vi "蓝牙串口接受.vi"() -> ()   [LabVIEW 2023]
uses:
  <vilib>/Instr/_visa.llb/VISA Flush IO Buffer Mask.ctl
  <vilib>/Instr/_visa.llb/VISA Configure Serial Port (Instr).vi
panel:
  out "同道2波形":u32(graph)
  out "通道1波形":u32(graph)
  in  "write_buffer":string
  in  "发送按钮":bool
  out "ReadBuffer":string
  out "读取返回数":u32
  in  "serial":refnum<visa-resource-name> caption="VISA资源名称"
  in  "串口开关":bool
  out "串口状态":bool
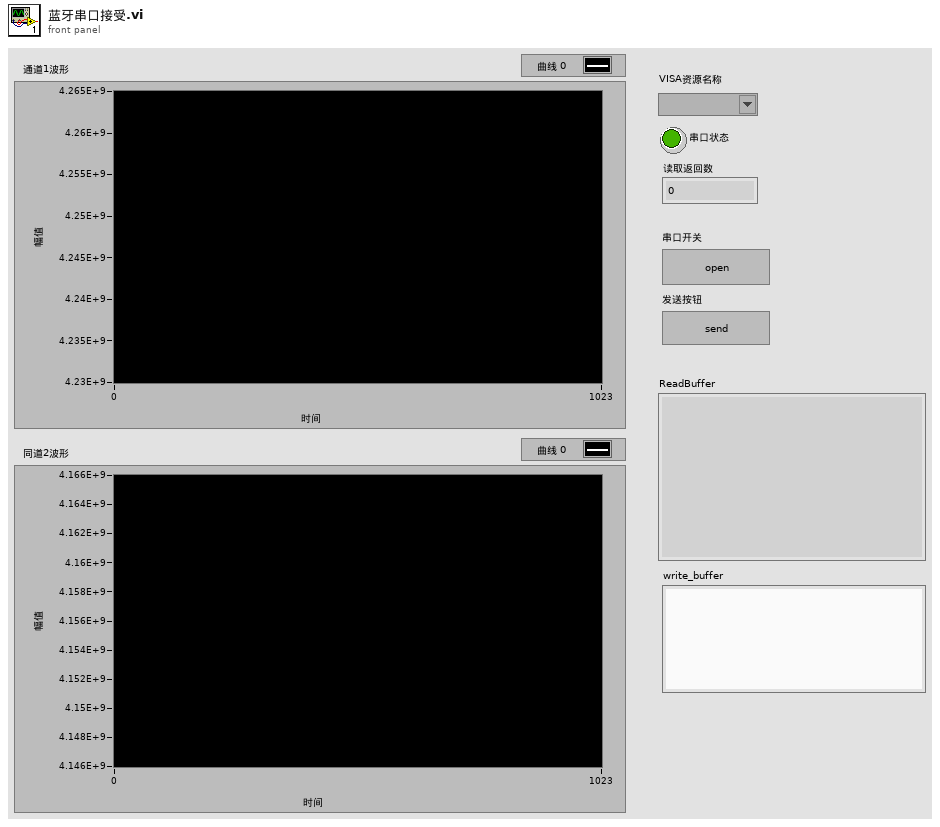
[diagram p1: front panel]
types:
  T1 = enum16{"nohead", "get_BB", "get_AA", "get_crc", "get_cnt"}
  T2 = cluster{"rx_finish":bool, "data_len":u8, "data":u8[], "head":enum16{"nohead", "get_BB", "get_AA", "get_crc", "get_cnt"}, "CRC":u8, "cnt":u8, "rx_len":u8}
  T3 = typedef "状态机控件.ctl" = enum16{"init_state", "main_state", "uart_receive_state", "stop_state"}
  T4 = typedef "VISA Flush IO Buffer Mask.ctl" = u16
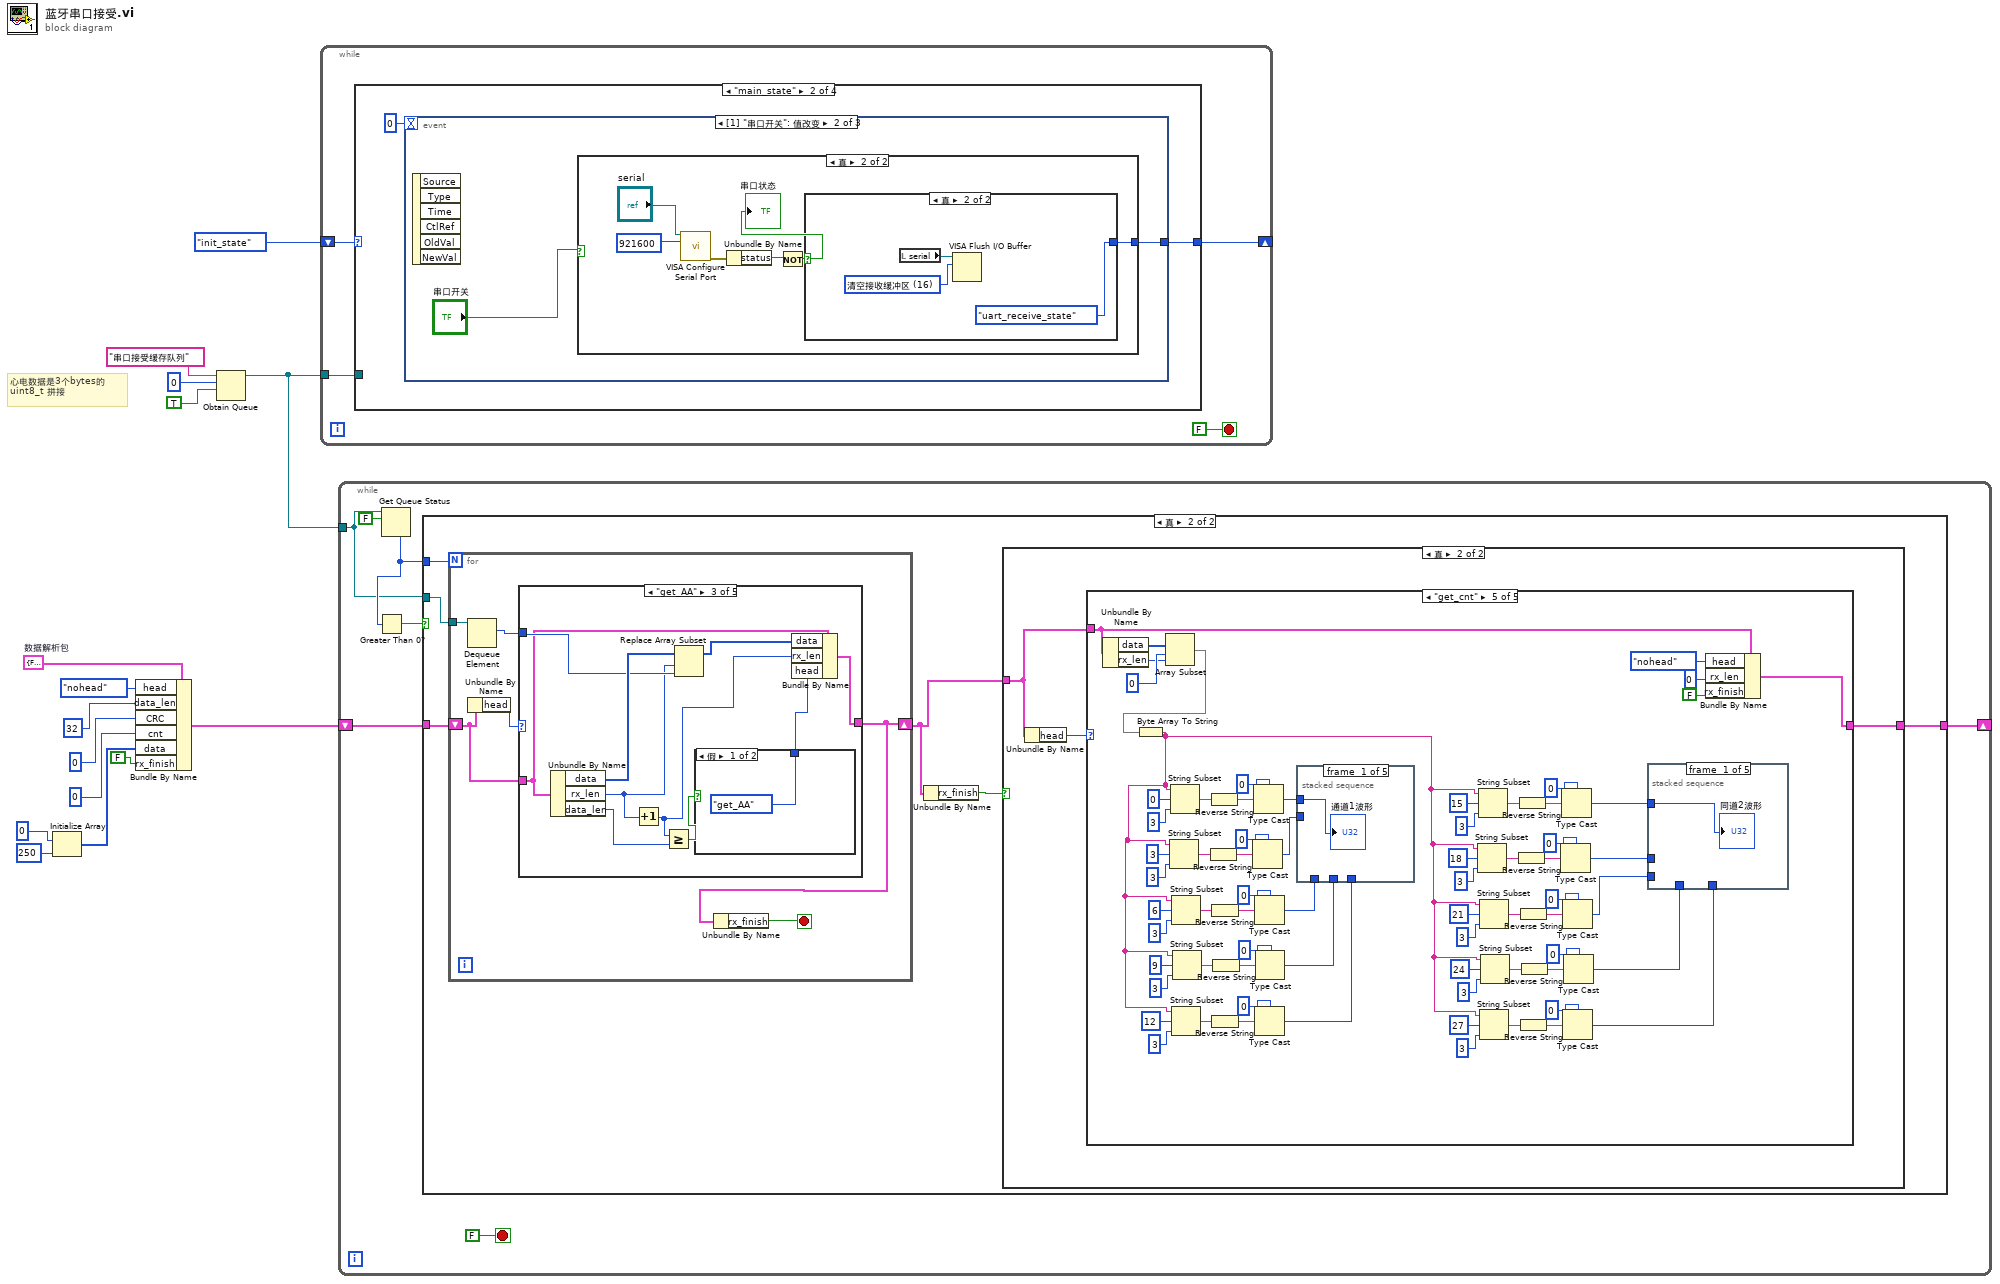
[diagram p0: block diagram]
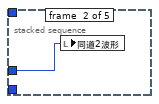
[diagram p8: hidden frame]
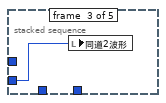
[diagram p9: hidden frame]
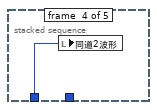
[diagram p10: hidden frame]
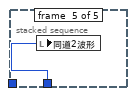
[diagram p11: hidden frame]
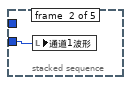
[diagram p12: hidden frame]
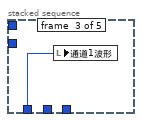
[diagram p13: hidden frame]
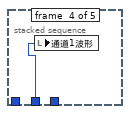
[diagram p14: hidden frame]
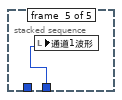
[diagram p15: hidden frame]
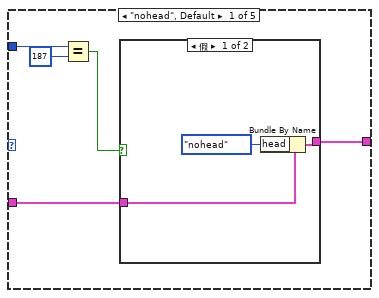
[diagram p16: hidden frame]
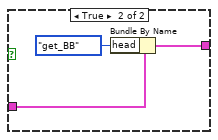
[diagram p17: hidden frame]
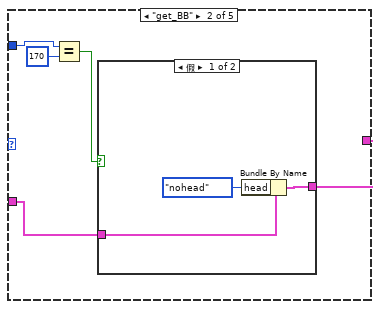
[diagram p18: hidden frame]
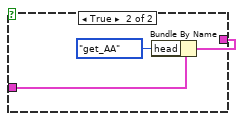
[diagram p19: hidden frame]
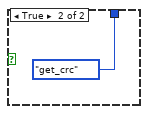
[diagram p20: hidden frame]
diagram:
  w11 = T2 {"rx_finish"=FALSE, "data_len"=0, "data"=[], "head"=enum."nohead", "CRC"=0, "cnt"=0, "rx_len"=0}  # 数据解析包
  # "心电数据是3个bytes的\nuint8_t 拼接"
  n1 = Initialize Array(u8 0 ("元素"), 250 ("维数大小")) -> (w4:u8[])
  n2 = Bundle By Name(cluster=w11, "head"=T1."nohead", "data_len"=u8 32, "CRC"=u8 0, "cnt"=u8 0 ("data_cnt"), "data"=w4, "rx_finish"=FALSE) -> (w10:T2)
  n3 = Obtain Queue(name (unnamed)="串口接受缓存队列" ("名称（未命名）"), element data type=u8 0, create if not found? (T)=TRUE ("如未找到则创建？(T)")) -> (queue out=w2:refnum<queue>)  [unwired: 2 in, 2 out]
  n4 = while {
    shift-right: [w19] -> _
    shift-left: 状态机控件."init_state" ("枚举") -> [w18]
    tunnel: w2 -> [w17]
    stop <- FALSE stop-if-true
    n5 = case shown="\"main_state\"" w18 {
      tunnel: [状态机控件."main_state" ("枚举") w27 w62 状态机控件."stop_state" ("枚举")] -> w19
      tunnel: w17 -> [_ _ w57 _]
      frame "init_state", Default {
        n6 = local write "write_buffer"("" ("write_buffer")) -> ()
        n7 = local write "ReadBuffer"("" ("ReadBuffer")) -> ()
        n8 = local write "串口开关"(FALSE ("串口状态")) -> ()
        n9 = local write "串口状态"(FALSE ("串口状态")) -> ()
        n10 = global write "全局变量1.vi" "while开关"(FALSE ("全局变量while开关")) -> ()
      }
      frame "main_state" {
        n11 = event shown="[1] \"串口开关\": 值改变" {
          selector: _ -> [_ _ _]
          dyn-events: _ -> [_ _ _]
          timeout: 0 -> [_ _ _]
          tunnel: [w29 w32 w50] -> w27
          event Timeout {
            n12 = event-data() -> ()  [unwired: 1 in, 3 out]
            n13 = local read "串口状态"() -> (w28:bool)
            n14 = case shown="假" w28 {
              tunnel: [状态机控件."main_state" ("枚举") 状态机控件."uart_receive_state" ("枚举")] -> w29
              frame False {
              }
              frame True {
              }
            }
          }
          event "串口开关": Value Change {
            n15 = event-data() -> ()  [unwired: 1 in, 6 out]
            n16 = case shown="真" "串口开关" {
              tunnel: [状态机控件."main_state" ("枚举") w37] -> w32
              frame False {
                # "关闭串口"
                n17 = local write "串口状态"(FALSE ("串口状态")) -> ()
                n18 = local read "serial"() -> (w35:refnum<visa-resource-name>)
                n19 = VISA Close(VISA resource name=w35) -> ()  [unwired: 1 in, 1 out]
              }
              frame True {
                n20 = call-poly "VISA Configure Serial Port"("VISA resource name"="serial", "baud rate (9600)"=u32 921600) -> ("error out"=w40:errorcluster)  [unwired: 12 in, 1 out]
                n21 = Unbundle By Name(w40) -> ("status"=w39:bool)
                n22 = Not(x=w39) -> (.not. x?=w38:bool)
                "串口状态" <- w38
                n23 = case shown="真" w38 {
                  tunnel: [状态机控件."main_state" ("枚举") 状态机控件."uart_receive_state" ("枚举")] -> w37
                  frame False {
                    n24 = local write "串口开关"(FALSE ("串口状态")) -> ()
                    n25 = One Button Dialog(message="串口打开失败" ("消息")) -> ()  [unwired: 1 in, 1 out]
                  }
                  frame True {
                    w46 = T4 16 items=["清空接收缓冲区"=16, "向设备写入传输缓冲区"=32, "清空接收缓冲区（无I/O）"=64, "清空传输缓冲区"=128] ("Mask")
                    n26 = local read "serial"() -> (w47:refnum<visa-resource-name>)
                    n27 = VISA Flush I/O Buffer(VISA resource name=w47, mask (16)=w46) -> ()  [unwired: 1 in, 2 out]
                  }
                }
              }
            }
          }
          event "发送按钮": Value Change {
            n28 = event-data() -> ()  [unwired: 1 in, 6 out]
            n29 = local read "串口状态"() -> (w49:bool)
            n30 = case shown="真" w49 {
              tunnel: [状态机控件."main_state" ("枚举") 状态机控件."uart_receive_state" ("枚举")] -> w50
              frame False {
                n31 = One Button Dialog(message="打开串口后在发送" ("消息")) -> ()  [unwired: 1 in, 1 out]
              }
              frame True {
                n32 = global write "全局变量1.vi" "while开关"(FALSE ("while开关")) -> ()
                n33 = local read "serial"() -> (w56:refnum<visa-resource-name>)
                n34 = VISA Write(VISA resource name=w56, write buffer="write_buffer") -> ()  [unwired: 1 in, 3 out]
              }
            }
          }
        }
      }
      frame "uart_receive_state" {
        n35 = local read "serial"() -> (w58:refnum<visa-resource-name>)
        n36 = property class="Instr"(reference=w58) -> (reference out=w60:refnum<visa-resource-name>, "Serial Settings:Number of Bytes at Serial Port"=w59:u32)  [unwired: 1 in, 1 out]
        n37 = Greater Than 0?(x=w59) -> (x > 0?=w61:bool)
        n38 = case shown="真" w61 {
          tunnel: [状态机控件."main_state" ("枚举") 状态机控件."main_state" ("枚举")] -> w62
          tunnel: w60 -> [_ w69]
          tunnel: w59 -> [_ w68]
          tunnel: w57 -> [_ w64]
          frame False {
          }
          frame True {
            # "注意点：for循环无法使用数组\n记住要关闭隧道索引"
            n39 = VISA Read(VISA resource name=w69, byte count=w68) -> (read buffer=w67:string)  [unwired: 1 in, 3 out]
            "ReadBuffer" <- w67
            n40 = String To Byte Array(string=w67) -> (unsigned byte array=w65:u8[])
            n41 = Array Size(array=w65) -> (size(s)=w66:i32)
            n42 = for {
              N: w66 -> [_]
              tunnel: w65 -> [w74]
              tunnel: w64 -> [w72]
              i -> [w73]
              # "队列数据通信 - > 队列操作\n\n先将串口读取到的数据存入队列"
              n43 = Index Array(array=w74, index=w73) -> (element=w71:u8)
              n44 = Enqueue Element(queue=w72, element=w71) -> ()  [unwired: 2 in, 3 out]
            }
            "读取返回数" <- w68
          }
        }
      }
      frame "stop_state" {
      }
    }
  }
  n45 = while {
    shift-right: [w78] -> _
    shift-left: w10 -> [w79]
    tunnel: w2 -> [w80]
    stop <- FALSE stop-if-true
    n46 = Get Queue Status(queue=w80, return elements? (F)=FALSE ("返回元素？(F)")) -> (# elements in queue=w81:i32)  [unwired: 1 in, 7 out]
    n47 = Greater Than 0?(x=w81) -> (x > 0?=w82:bool)
    n48 = case shown="真" w82 {
      tunnel: w81 -> [_ w89]
      tunnel: w80 -> [_ w88]
      tunnel: w79 -> [w83 w87]
      tunnel: [w83 w85] -> w78
      frame False {
      }
      frame True {
        n49 = for {
          N: w89 -> [_]
          tunnel: w88 -> [w183]
          shift-right: [w179] -> w84
          shift-left: w87 -> [w180]
          stop <- w178 stop-if-true
          n50 = Dequeue Element(queue=w183) -> (element=w181:u8)  [unwired: 2 in, 3 out]
          n51 = Unbundle By Name(w180) -> ("head"=w182:T1)
          n52 = case shown="\"get_AA\"" w182 {
            tunnel: w181 -> [w188 w198 w214 w220 w224]
            tunnel: w180 -> [w185 w197 w207 w221 w225]
            tunnel: [w184 w196 w206 w218 w223] -> w179
            frame "nohead", Default {
              n53 = Equal?(x=w188, y=u8 187) -> (x = y?=w186:bool)
              n54 = case shown="假" w186 {
                tunnel: w185 -> [w191 w194]
                tunnel: [w190 w193] -> w184
                frame False {
                  n55 = Bundle By Name(cluster=w191, "head"=T1."nohead") -> (w190:T2)
                }
                frame True {
                  n56 = Bundle By Name(cluster=w194, "head"=T1."get_BB") -> (w193:T2)
                }
              }
            }
            frame "get_BB" {
              n57 = Equal?(x=w198, y=u8 170) -> (x = y?=w195:bool)
              n58 = case shown="假" w195 {
                tunnel: w197 -> [w202 w205]
                tunnel: [w201 w204] -> w196
                frame False {
                  n59 = Bundle By Name(cluster=w202, "head"=T1."nohead") -> (w201:T2)
                }
                frame True {
                  n60 = Bundle By Name(cluster=w205, "head"=T1."get_AA") -> (w204:T2)
                }
              }
            }
            frame "get_AA" {
              n61 = Unbundle By Name(w207) -> ("data"=w215:u8[], "rx_len"=w213:u8, "data_len"=w212:u8)
              n62 = Increment(x=w213) -> (x+1=w210:u8)
              n63 = Greater Or Equal?(x=w210, y=w212) -> (x >= y?=w211:bool)
              n64 = Replace Array Subset(array=w215, new element=w214, index=w213) -> (w209:u8[])
              n65 = case shown="假" w211 {
                tunnel: [T1."get_AA" ("head") T1."get_crc" ("head")] -> w208
                frame False {
                }
                frame True {
                }
              }
              n66 = Bundle By Name(cluster=w207, "data"=w209, "rx_len"=w210, "head"=w208) -> (w206:T2)
            }
            frame "get_crc" {
              n67 = Bundle By Name(cluster=w221, "head"=T1."get_cnt", "CRC"=w220) -> (w218:T2)
            }
            frame "get_cnt" {
              n68 = Bundle By Name(cluster=w225, "rx_finish"=TRUE, "head"=T1."get_cnt", "cnt"=w224) -> (w223:T2)
            }
          }
          n69 = Unbundle By Name(w179) -> ("rx_finish"=w178:bool)
        }
        n70 = Unbundle By Name(w84) -> ("rx_finish"=w86:bool)
        n71 = case shown="真" w86 {
          tunnel: [w90 w92] -> w85
          tunnel: w84 -> [w90 w91]
          frame False {
          }
          frame True {
            n72 = Unbundle By Name(w91) -> ("head"=w93:T1)
            n73 = case shown="\"get_cnt\"" w93 {
              tunnel: [w94 w95 w96 w97 w98] -> w92
              tunnel: w91 -> [w94 w95 w96 w97 w102]
              frame "nohead", Default {
              }
              frame "get_BB" {
              }
              frame "get_AA" {
              }
              frame "get_crc" {
              }
              frame "get_cnt" {
                n74 = Unbundle By Name(w102) -> ("data"=w167:u8[], "rx_len"=w165:u8)
                n75 = Array Subset(array=w167, index=0 ("索引"), length=w165) -> (w164:u8[])
                n76 = Byte Array To String(unsigned byte array=w164) -> (string=w108:string)
                n77 = String Subset(string=w108, offset (0)=u32 3 ("偏移量(0)"), length (rest)=u32 3 ("长度（剩余）")) -> (substring=w149:string)
                n78 = String Subset(string=w108, offset (0)=u32 0 ("偏移量(0)"), length (rest)=u32 3 ("长度（剩余）")) -> (substring=w160:string)
                n79 = String Subset(string=w108, offset (0)=u32 6 ("偏移量(0)"), length (rest)=u32 3 ("长度（剩余）")) -> (substring=w143:string)
                n80 = String Subset(string=w108, offset (0)=u32 12 ("偏移量(0)"), length (rest)=u32 3 ("长度（剩余）")) -> (substring=w141:string)
                n81 = String Subset(string=w108, offset (0)=u32 9 ("偏移量(0)"), length (rest)=u32 3 ("长度（剩余）")) -> (substring=w145:string)
                n82 = Reverse String(1:w149) -> (0:w155:string)
                n83 = Reverse String(1:w160) -> (0:w161:string)
                n84 = Reverse String(1:w143) -> (0:w152:string)
                n85 = Reverse String(1:w141) -> (0:w140:string)
                n86 = Reverse String(1:w145) -> (0:w146:string)
                n87 = Type Cast(type=u32 0, x=w155) -> (*(type *) &x=w137:u32)
                n88 = Type Cast(type=u32 0, x=w161) -> (*(type *) &x=w158:u32)
                n89 = Type Cast(type=u32 0, x=w152) -> (*(type *) &x=w136:u32)
                n90 = Type Cast(type=u32 0, x=w140) -> (*(type *) &x=w134:u32)
                n91 = Type Cast(type=u32 0, x=w146) -> (*(type *) &x=w135:u32)
                n92 = stacked-sequence {
                  tunnel: w158 -> [w173 _ _ _ _]
                  tunnel: w137 -> [_ w174 _ _ _]
                  tunnel: w136 -> [_ _ w175 _ _]
                  tunnel: w135 -> [_ _ _ w176 _]
                  tunnel: w134 -> [_ _ _ _ w177]
                  frame #0 {
                    "通道1波形" <- w173
                  }
                  frame #1 {
                    n93 = local write "通道1波形"(w174) -> ()
                  }
                  frame #2 {
                    n94 = local write "通道1波形"(w175) -> ()
                  }
                  frame #3 {
                    n95 = local write "通道1波形"(w176) -> ()
                  }
                  frame #4 {
                    n96 = local write "通道1波形"(w177) -> ()
                  }
                }
                n97 = String Subset(string=w108, offset (0)=u32 18 ("偏移量(0)"), length (rest)=u32 3 ("长度（剩余）")) -> (substring=w120:string)
                n98 = String Subset(string=w108, offset (0)=u32 15 ("偏移量(0)"), length (rest)=u32 3 ("长度（剩余）")) -> (substring=w130:string)
                n99 = String Subset(string=w108, offset (0)=u32 21 ("偏移量(0)"), length (rest)=u32 3 ("长度（剩余）")) -> (substring=w114:string)
                n100 = String Subset(string=w108, offset (0)=u32 27 ("偏移量(0)"), length (rest)=u32 3 ("长度（剩余）")) -> (substring=w112:string)
                n101 = String Subset(string=w108, offset (0)=u32 24 ("偏移量(0)"), length (rest)=u32 3 ("长度（剩余）")) -> (substring=w116:string)
                n102 = Reverse String(1:w120) -> (0:w126:string)
                n103 = Reverse String(1:w130) -> (0:w131:string)
                n104 = Reverse String(1:w114) -> (0:w123:string)
                n105 = Reverse String(1:w112) -> (0:w111:string)
                n106 = Reverse String(1:w116) -> (0:w117:string)
                n107 = Type Cast(type=u32 0, x=w126) -> (*(type *) &x=w106:u32)
                n108 = Type Cast(type=u32 0, x=w131) -> (*(type *) &x=w107:u32)
                n109 = Type Cast(type=u32 0, x=w123) -> (*(type *) &x=w105:u32)
                n110 = Type Cast(type=u32 0, x=w111) -> (*(type *) &x=w103:u32)
                n111 = Type Cast(type=u32 0, x=w117) -> (*(type *) &x=w104:u32)
                n112 = stacked-sequence {
                  tunnel: w107 -> [w168 _ _ _ _]
                  tunnel: w106 -> [_ w169 _ _ _]
                  tunnel: w105 -> [_ _ w170 _ _]
                  tunnel: w104 -> [_ _ _ w171 _]
                  tunnel: w103 -> [_ _ _ _ w172]
                  frame #0 {
                    "同道2波形" <- w168
                  }
                  frame #1 {
                    n113 = local write "同道2波形"(w169) -> ()
                  }
                  frame #2 {
                    n114 = local write "同道2波形"(w170) -> ()
                  }
                  frame #3 {
                    n115 = local write "同道2波形"(w171) -> ()
                  }
                  frame #4 {
                    n116 = local write "同道2波形"(w172) -> ()
                  }
                }
                n117 = Bundle By Name(cluster=w102, "head"=T1."nohead", "rx_len"=u8 0, "rx_finish"=FALSE) -> (w98:T2)
              }
            }
          }
        }
      }
    }
  }
